vi "Variables Write for Position Control.vi"(4 "Reference Phase":dbl, 5 "Measured Position":dbl[](array[numeric]), 6 "Reference X,Y":dbl[](array[numeric]), 7 "Reference Tension":dbl[](array[numeric]), 8 "Motors Configuration":dbl[][](array[numeric]), 9 "Ellipse Length":dbl[](array[numeric]), 10 "Jacobian":dbl[][](array[numeric]), 11 "Measured Phase":dbl) -> ()   [LabVIEW 2021]
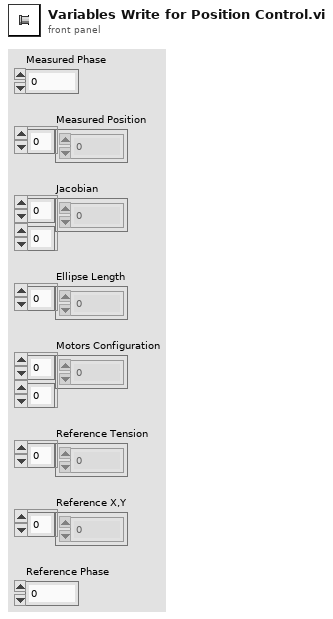
[diagram p1: front panel]
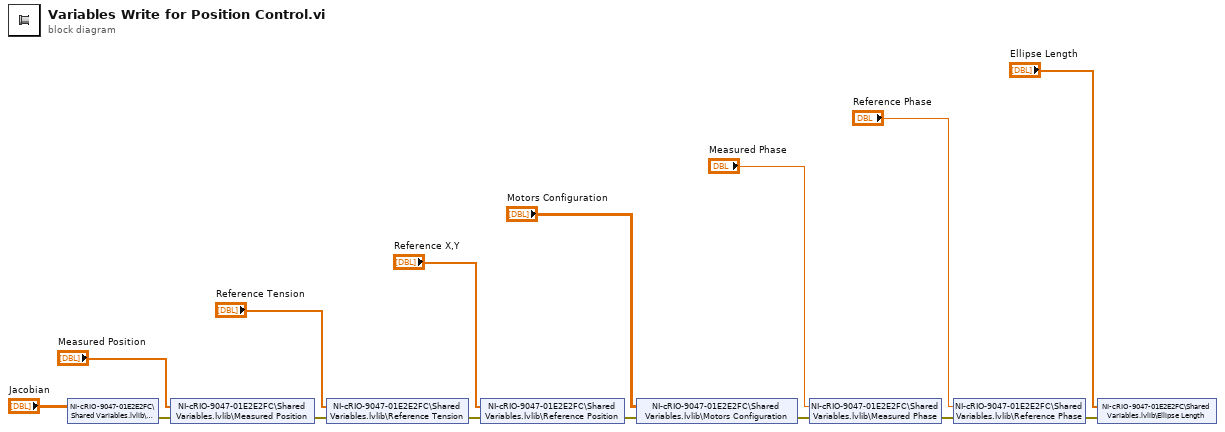
[diagram p0: block diagram]
diagram:
  n1 = shared-variable "NI-cRIO-9047-01E2E2FC\\Shared Variables.lvlib\\Jacobian"("Jacobian") -> (error out=w4:errorcluster)  [unwired: 1 in]
  n2 = shared-variable "NI-cRIO-9047-01E2E2FC\\Shared Variables.lvlib\\Measured Position"("Measured Position", error in=w4) -> (error out=w3:errorcluster)
  n3 = shared-variable "NI-cRIO-9047-01E2E2FC\\Shared Variables.lvlib\\Reference Tension"("Reference Tension", error in=w3) -> (error out=w9:errorcluster)
  n4 = shared-variable "NI-cRIO-9047-01E2E2FC\\Shared Variables.lvlib\\Reference Position"("Reference X,Y", error in=w9) -> (error out=w2:errorcluster)
  n5 = shared-variable "NI-cRIO-9047-01E2E2FC\\Shared Variables.lvlib\\Motors Configuration"("Motors Configuration", error in=w2) -> (error out=w1:errorcluster)
  n6 = shared-variable "NI-cRIO-9047-01E2E2FC\\Shared Variables.lvlib\\Measured Phase"("Measured Phase", error in=w1) -> (error out=w8:errorcluster)
  n7 = shared-variable "NI-cRIO-9047-01E2E2FC\\Shared Variables.lvlib\\Reference Phase"("Reference Phase", error in=w8) -> (error out=w7:errorcluster)
  n8 = shared-variable "NI-cRIO-9047-01E2E2FC\\Shared Variables.lvlib\\Ellipse Length"("Ellipse Length", error in=w7) -> ()  [unwired: 1 out]
